vi "Servo_Controller.vi"(4 "error in (no error)":errorcluster, 5 "PWM Ref In":T1, 6 "null offset":bool, 7 "position [%FS]":dbl(slide) scale=-200.0..200.0) -> (0 "error out":errorcluster, 1 "duty cycle [%]":dbl, 2 "pulse width [ms]":dbl=1.5, 3 "offset [%FS]":dbl)   [LabVIEW 2017]
uses:
  <vilib>/myRIO/Instrument Drivers/Onboard IO/PWM/typedefs/PWM Reference.ctl
  <vilib>/myRIO/Common/Instrument Driver Framework/Utilities/typedefs/myRIO Generic Hardware Reference.ctl
  <vilib>/myRIO/Common/Instrument Driver Framework/Utilities/typedefs/Hardware Version Enum.ctl
  <vilib>/myRIO/Common/Instrument Driver Framework/Utilities/typedefs/myRIO v1.0 Reference.ctl
  <vilib>/myRIO/Common/Instrument Driver Framework/Utilities/typedefs/Generic FPGA Reference.ctl
  <vilib>/myRIO/Common/Instrument Driver Framework/myRIO v1.0/PWM/typedefs/PWM Channels Enum.ctl
  <vilib>/myRIO/Instrument Drivers/Onboard IO/PWM/typedefs/PWM Configuration.ctl
  <vilib>/Utility/error.llb/Error Cluster From Error Code.vi
  <vilib>/myRIO/Common/Instrument Driver Framework/myRIO v1.0/PWM/vis/myRIO v1.0 Write PWM.vi
  <vilib>/myRIO/Instrument Drivers/Onboard IO/PWM/PWM.lvlib
panel:
  in  "PWM Ref In 2":T1
  out "Pre-Set Frequency":dbl
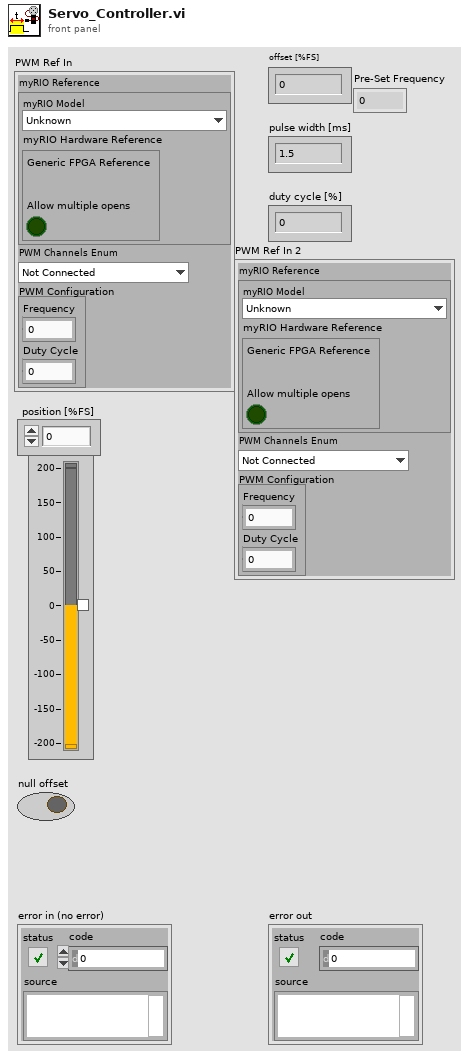
[diagram p1: front panel]
types:
  T1 = typedef "PWM.lvlib/PWM Reference.ctl" = cluster{"myRIO Reference":T2, "PWM Channels Enum":T6, "PWM Configuration":T7}
  T2 = typedef "myRIO Generic Hardware Reference.ctl" = cluster{"myRIO Model":T3, "myRIO Hardware Reference":T4}
  T3 = typedef "Hardware Version Enum.ctl" = enum16{"Unknown", "myRIO-1900", "myRIO-1950", "roboRIO", "NI ELVIS RIO CM"}
  T4 = typedef "myRIO v1.0 Reference.ctl" = cluster{"Generic FPGA Reference":T5, "Allow multiple opens":bool}
  T5 = typedef "Generic FPGA Reference.ctl" = refnum<k20>
  T6 = typedef "PWM Channels Enum.ctl" = enum16{"Not Connected", "C/PWM0", "C/PWM1", "A/PWM0", "A/PWM1", "A/PWM2", "B/PWM0", "B/PWM1", "B/PWM2", "PWM/PWM0", "PWM/PWM1", "PWM/PWM2", "PWM/PWM3", "PWM/PWM4", "PWM/PWM5", "PWM/PWM6", "PWM/PWM7", "PWM/PWM8", "PWM/PWM9"}
  T7 = typedef "PWM.lvlib/PWM Configuration.ctl" = cluster{"Frequency":dbl, "Duty Cycle":dbl}
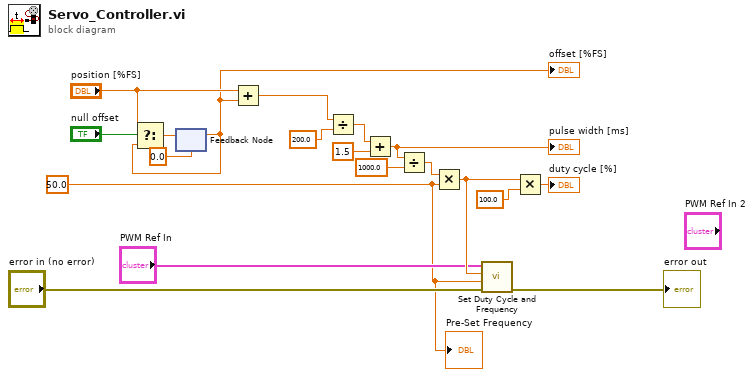
[diagram p0: block diagram]
diagram:
  w1 = 50.0 ("freq [Hz]")
  n1 = feedback #1(0.0 ("position [%FS]")) -> (w13:dbl)
  "offset [%FS]" <- w13
  n2 = Select(t="position [%FS]", s="null offset", f=w13) -> (s? t:f=w11:dbl)
  n3 = feedback-in #1(w11) -> ()
  n4 = Add(x="position [%FS]", y=w13) -> (x+y=w12:dbl)
  n5 = Divide(x=w12, y=200.0) -> (x/y=w4:dbl)
  n6 = Add(x=w4, y=1.5) -> (x+y=w6:dbl)
  "pulse width [ms]" <- w6
  n7 = Divide(x=w6, y=1000.0) -> (x/y=w14:dbl)
  n8 = Multiply(x=w14, y=w1) -> (x*y=w17:dbl)
  n9 = call <vilib>:"Set Duty Cycle and Frequency.vi"("error in (no error)"="error in (no error)", "Frequency [Hz]"=w1, "Duty Cycle"=w17, "PWM Ref In"="PWM Ref In") -> ("error out"=→"error out":errorcluster)  [unwired: 5 in, 1 out]
  n10 = Multiply(x=w17, y=100.0) -> (x*y=→"duty cycle [%]":dbl)
  "Pre-Set Frequency" <- w1
